vi "Write Current State Name.vi"(8 "error in (no error)":errorcluster, 10 "Current State Name":string, 11 "Command Processor in":refnum<class "Command Processor.lvclass">) -> (0 "error out":errorcluster, 3 "Command Processor out":refnum<class "Command Processor.lvclass">)   [LabVIEW 2013, in "Command Processor.lvlib" / "Command Processor.lvclass"]
uses:
  Command Processor.lvclass
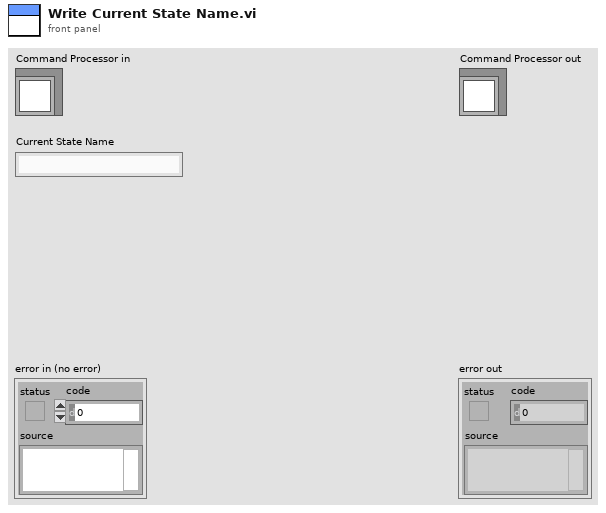
[diagram p1: front panel]
types:
  T1 = typedef "Command Processor.lvlib/Command Processor.lvclass/Command Processor Status.ctl" = cluster{"State Entry time":timestamp, "State Status":T2, "Command Processor Current State":string, "Command Status":T4}
  T2 = typedef "Current Previous State Status.ctl" = cluster{"Current State Status":T3, "Previous State Status":T3}
  T3 = typedef "State Status.ctl" = cluster{"State Name":string, "State Entry Time":timestamp, "State Exit Time":timestamp}
  T4 = typedef "Command Processor.lvlib/Command.lvlib/Command.lvclass/Command Status.ctl" = cluster{"Command Name":string, "Current State Status":T5, "Command Start Time":timestamp, "Command End Time":timestamp, "Previous State Status":T5}
  T5 = typedef "Command Processor.lvlib/Command.lvlib/Command.lvclass/State Status.ctl" = cluster{"State Name":string, "State Entry Time":timestamp, "State Exit Time":timestamp}
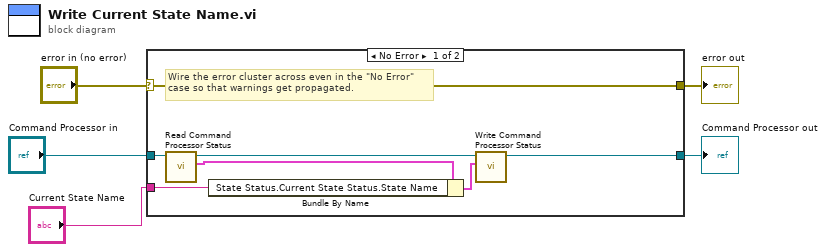
[diagram p0: block diagram]
diagram:
  n1 = case shown="No Error" "error in (no error)" {
    selector: "error in (no error)" -> [w12 w14]
    tunnel: [w12 w14] -> w4
    tunnel: [w10 w13] -> w2
    tunnel: "Command Processor in" -> [w11 w13]
    tunnel: "Current State Name" -> [w6 _]
    frame No Error {
      # "Wire the error cluster across even in the \"No Error\"\ncase so that warnings get propagated."
      n2 = call-dynamic "Read Command Processor Status.vi"("Command Processor in"=w11) -> ("Command Processor Status"=w8:T1, "Command Processor out"=w9:refnum<class "Command Processor.lvclass">)  [unwired: 8 in, 1 out]
      n3 = Bundle By Name(cluster=w8, "State Status.Current State Status.State Name"=w6) -> (w7:T1)
      n4 = call-dynamic "Write Command Processor Status.vi"("Command Processor Status"=w7, "Command Processor in"=w9) -> ("Command Processor out"=w10:refnum<class "Command Processor.lvclass">)  [unwired: 8 in, 1 out]
    }
    frame Error {
    }
  }
  "error out" <- w4
  "Command Processor out" <- w2
